vi "numeric to boolean.vi"(11 "Numeric":dbl) -> (0 "Boolean":bool)   [LabVIEW 2014]
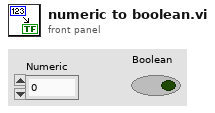
[diagram p1: front panel]
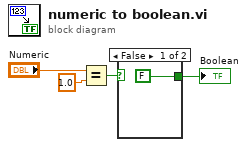
[diagram p0: block diagram]
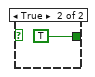
[diagram p2: hidden frame]
diagram:
  n1 = Equal?(x="Numeric", y=1.0) -> (x = y?=w4:bool)
  n2 = case shown="False" w4 {
    tunnel: [FALSE TRUE] -> w1
    frame False {
    }
    frame True {
    }
  }
  "Boolean" <- w1
